vi "Write.vi"(8 "Error in":errorcluster caption="Error in (no error)", 10 "dbl":dbl, 11 "DVR":T1) -> (0 "Error out":errorcluster, 3 "DVR(dup)":T1)   [LabVIEW 2020, in "DVR-Module.lvlib"]
uses:
  DVR-Module.lvlib
  DVR.ctl
  DataDef.ctl
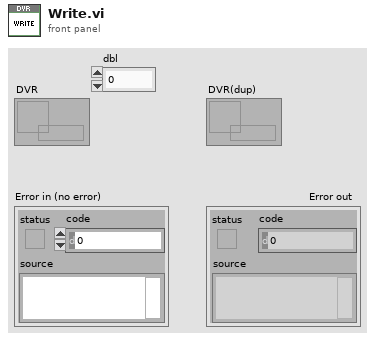
[diagram p1: front panel]
types:
  T1 = typedef "DVR-Module.lvlib/DVR.ctl" = refnum<data-value>
  T2 = typedef "DataDef.ctl" = cluster{"dbl":dbl}
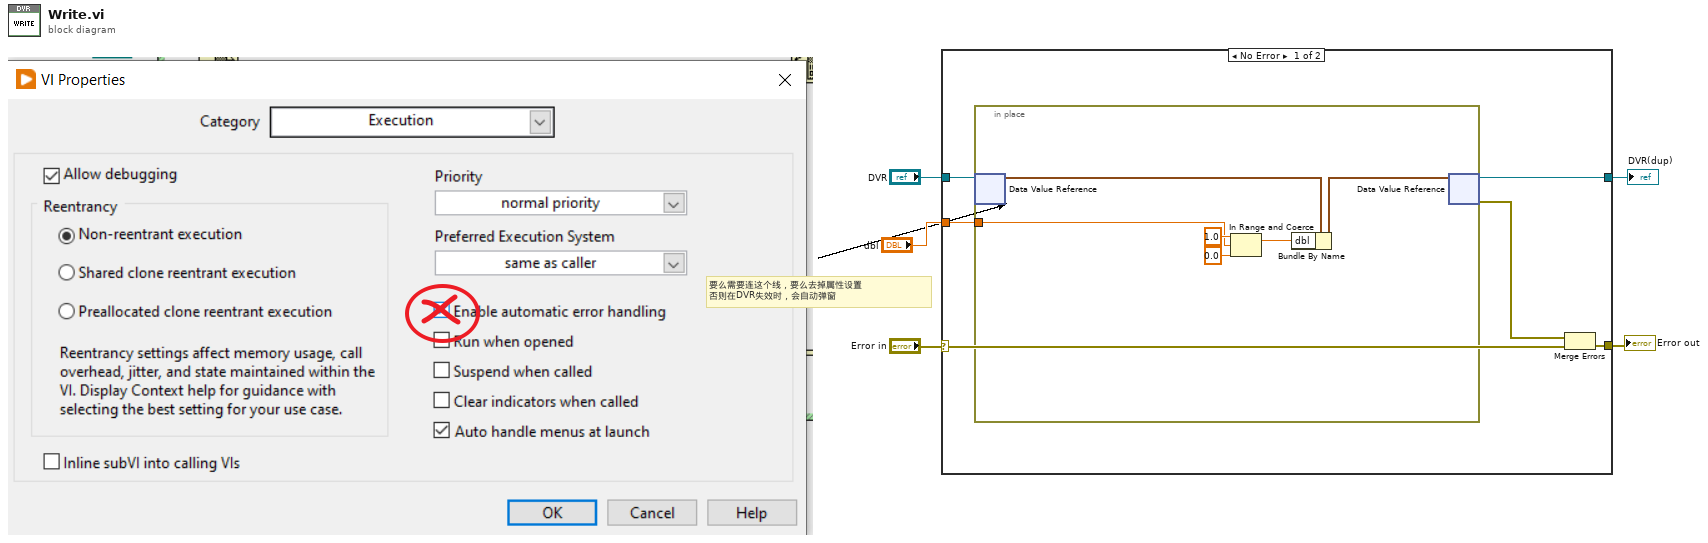
[diagram p0: block diagram]
diagram:
  # "要么需要连这个线，要么去掉属性设置\n否则在DVR失效时，会自动弹窗"
  n1 = case shown="No Error" "Error in" {
    selector: "Error in" -> [w7 w19]
    tunnel: "DVR" -> [w11 w18]
    tunnel: [w10 w18] -> w4
    tunnel: [w9 w19] -> w3
    tunnel: "dbl" -> [w6 _]
    frame No Error {
      n2 = in-place {
        in-place-border: w6 -> [w12]
        n3 = in-place-dvr #1(w11) -> (w17:T2)  [unwired: 1 out]
        n4 = In Range and Coerce(upper limit=1.0, x=w12, lower limit=0.0) -> (coerced(x)=w13:dbl)  [unwired: 1 out]
        n5 = Bundle By Name(cluster=w17, "dbl"=w13) -> (w16:T2)
        n6 = in-place-dvr #1(w16) -> (w10:T1, w8:errorcluster)
      }
      n7 = Merge Errors(w8, w7) -> (w9:errorcluster)
    }
    frame Error {
    }
  }
  "Error out" <- w3
  "DVR(dup)" <- w4
